vi "Get_RegGroup.vi"(8 "error in (no error)":errorcluster, 11 "IB_RegGroup in":refnum<class "IB_RegGroup.lvclass">) -> (0 "error out":errorcluster, 2 "data":T1, 3 "IB_RegGroup out":refnum<class "IB_RegGroup.lvclass">)   [LabVIEW 2020, in "IB_RegGroup.lvclass"]
uses:
  <vilib>/AppBuilder/IB_Classes/RegGroup/IB_RegGroup.lvclass
  <vilib>/AppBuilder/IB_Classes/RegGroup/IB_RegGroup.lvclass/IB_RegGroup.ctl
  <vilib>/AppBuilder/IB_Classes/RegData/IB_RegData.lvclass
  <vilib>/AppBuilder/IB_Classes/RegGroup/IB_RegGroup.ctl
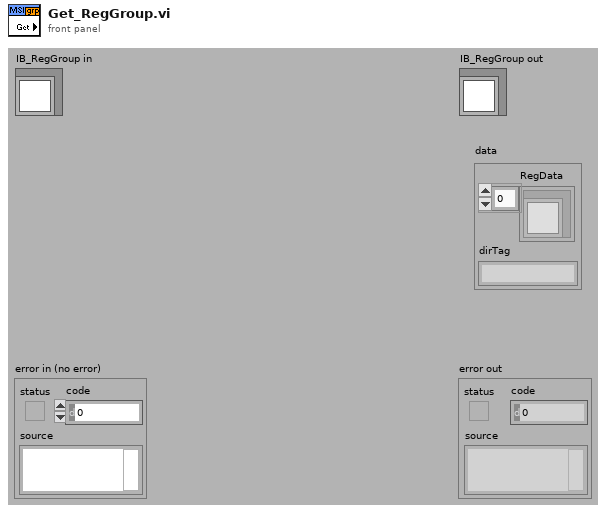
[diagram p1: front panel]
types:
  T1 = typedef "IB_RegGroup.ctl" = cluster{"RegData":refnum<class "IB_RegData.lvclass">[], "dirTag":string}
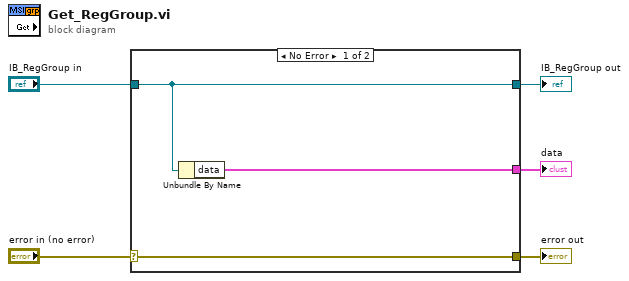
[diagram p0: block diagram]
diagram:
  n1 = case shown="No Error" "error in (no error)" {
    selector: "error in (no error)" -> [w8 w9]
    tunnel: [w8 w9] -> w4
    tunnel: [w7 w10] -> w2
    tunnel: "IB_RegGroup in" -> [w7 w10]
    tunnel: [w6 _] -> w1
    frame No Error {
      n2 = Unbundle By Name(w7) -> ("data"=w6:T1)
    }
    frame Error {
    }
  }
  "error out" <- w4
  "IB_RegGroup out" <- w2
  "data" <- w1
